vi "ZSLIM_OP100_LabelPrint.vi"(7 "Cluster":T1, 8 "errin":errorcluster) -> (0 "error out":errorcluster caption="errout")   [LabVIEW 2020]
uses:
  <vilib>/httpClient/POSTBuffer.vi
  <vilib>/httpClient/LabVIEWHTTPClient.lvlib
panel:
  out "body":string caption="corps"
  out "headers":string caption="en-têtes"
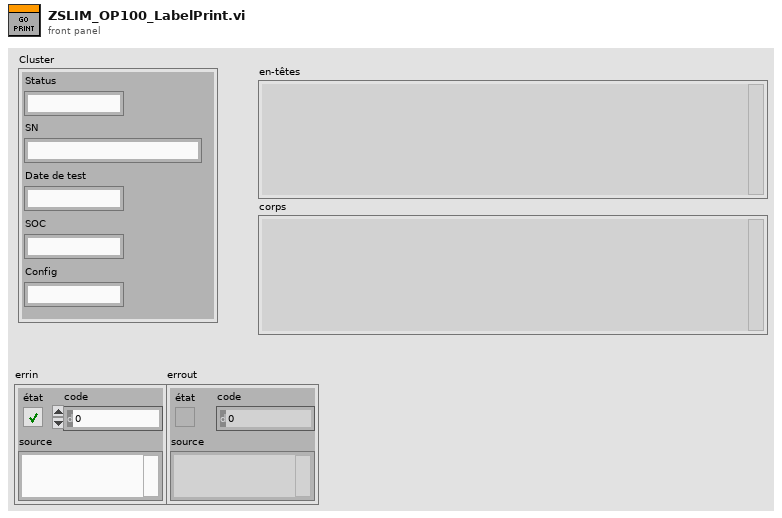
[diagram p1: front panel]
types:
  T1 = cluster{"Status":string, "SN":string, "Date de test":string, "SOC":string, "Config":string}
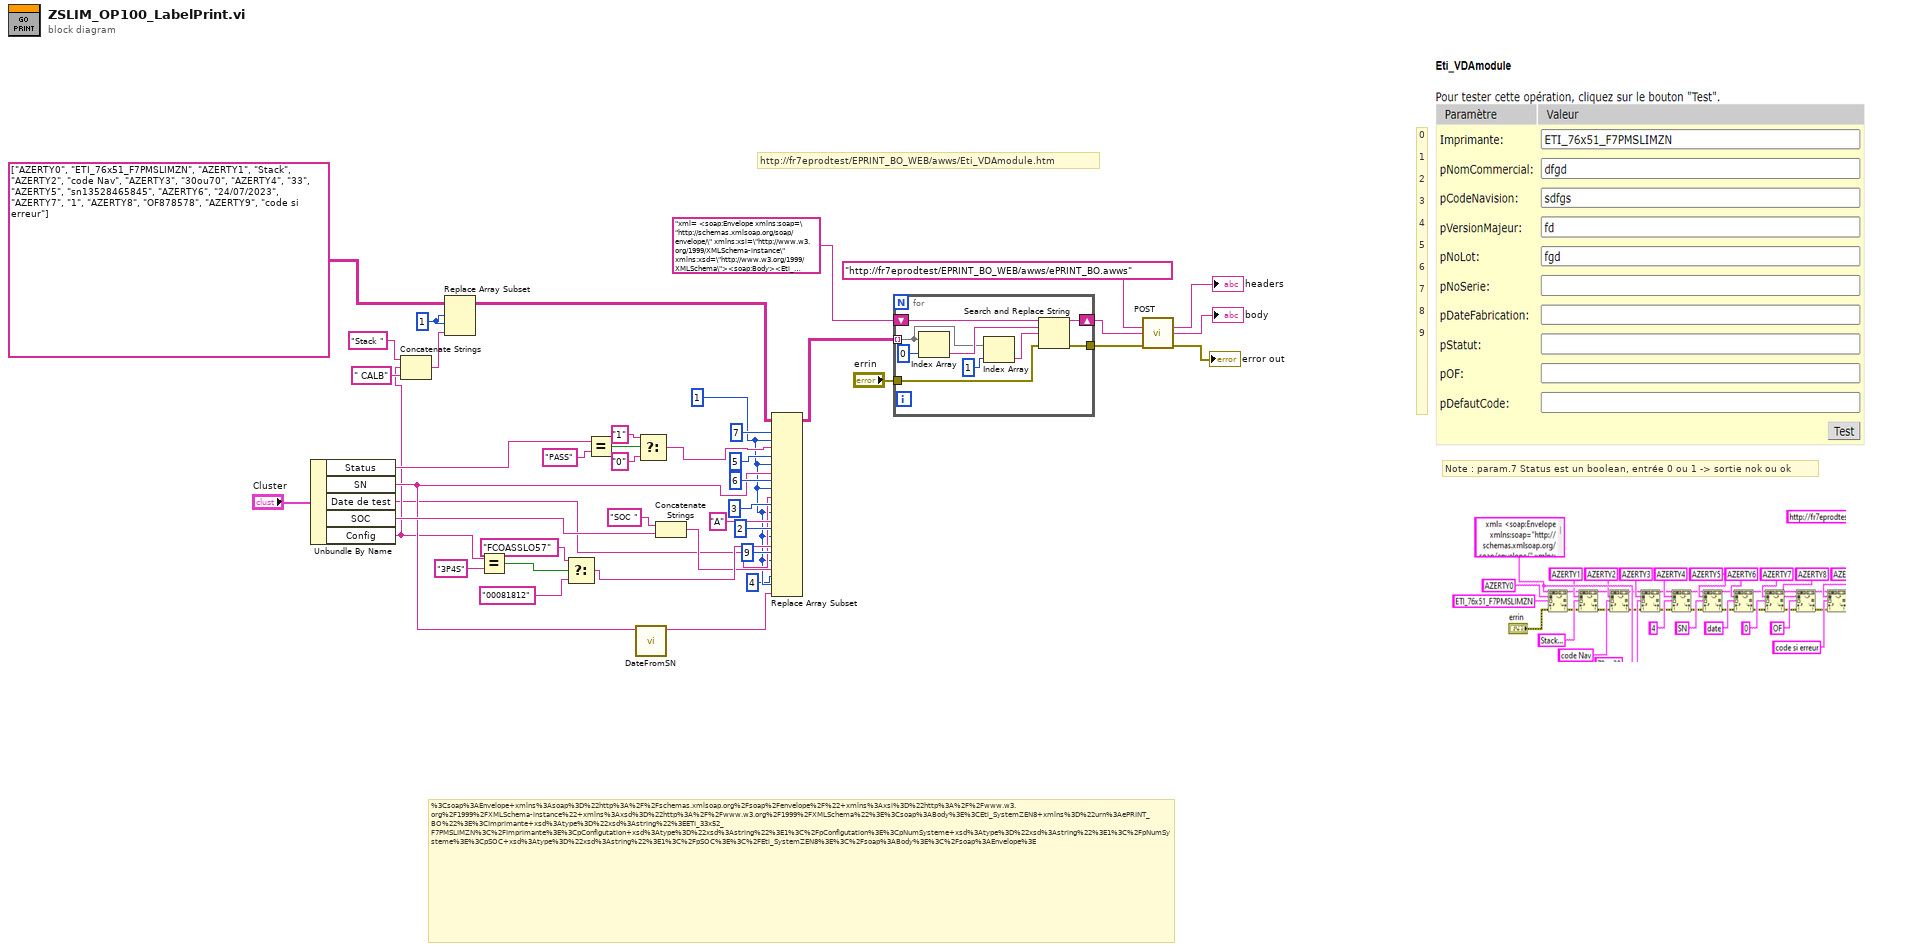
[diagram p0: block diagram]
diagram:
  w19 = 1 ("disabled index (col)")
  w2 = 1 ("disabled index (col)")
  # "http://fr7eprodtest/EPRINT_BO_WEB/awws/Eti_VDAmodule.htm"
  # "Note : param.7 Status est un boolean, entrée 0 ou 1 -> sortie nok ou ok"
  # "0\n\n1\n\n2\n\n3\n\n4\n\n5\n\n6\n\n7\n\n8\n\n9"
  # "%3Csoap%3AEnvelope+xmlns%3Asoap%3D%22http%3A%2F%2Fschemas.xmlsoap.org%2Fsoap%2Fenvelope%2F%22+xmlns%3Axsi%3D%22http%3A%2F%2Fwww.w3.org%2F1999%2FXMLSchema-instance%22+xmlns%3Axsd%3D%22http%3A%2F%2Fwww.w3.org%2F1999%2FXMLSchema%22%3E%3Csoap%3ABody%3E%3CEti_SystemZEN8+xmlns%3D%22urn%3AePRINT_BO%22%3E%3CImprimante+xsd%3Atype%3D%22xsd%3Astring%22%3EETI_33x52_F7PMSLIMZN%3C%2FImprimante%3E%3CpConfigutation+xsd%3Atype%3D%22xsd%3Astring%22%3E1%3C%2FpConfigutation%3E%3CpNumSysteme+xsd%3Atype%3D%22xsd%3Astring%22%3E1%3C%2FpNumSysteme%3E%3CpSOC+xsd%3Atype%3D%22xsd%3Astring%22%3E1%3C%2FpSOC%3E%3C%2FEti_SystemZEN8%3E%3C%2Fsoap%3ABody%3E%3C%2Fsoap%3AEnvelope%3E"
  n1 = Unbundle By Name("Cluster") -> ("Status"=w21:string, "SN"=w15:string, "Date de test"=w4:string, "SOC"=w20:string, "Config"=w13:string)
  n2 = Concatenate Strings("Stack " ("string"), w13, " CALB" ("string")) -> (w16:string)
  n3 = Replace Array Subset(array=string[][] [["AZERTY0", "ETI_76x51_F7PMSLIMZN"], ["AZERTY1", "Stack"], ["AZERTY2", "code Nav"], ["AZERTY3", "30ou70"], ["AZERTY4", "33"], ["AZERTY5", "sn13528465845"], ["AZERTY6", "24/07/2023"], ["AZERTY7", "1"], ["AZERTY8", "OF878578"], ["AZERTY9", "code si erreur"]], new element=w16, index (row)=w19, index (col)=w19) -> (w23:string[][])
  n4 = Equal?(x=w13, y="3P4S") -> (x = y?=w11:bool)
  n5 = Select(t="FCOASSLO57" ("y"), s=w11, f="00081812" ("y")) -> (s? t:f=w8:string)
  n6 = Equal?(x=w21, y="PASS") -> (x = y?=w34:bool)
  n7 = call "DateFromSN.vi"("SN"=w15) -> ("Date de fab"=w3:string)  [unwired: 10 in]
  n8 = Select(t="1" ("y"), s=w34, f="0") -> (s? t:f=w28:string)
  n9 = Concatenate Strings("SOC " ("string"), w20) -> (w5:string)
  n10 = Replace Array Subset(array=w23, new element #1=w28, index (row) #1=7 ("index (row)"), index (col) #1=w2, new element #2=w15, index (row) #2=5 ("disabled index (row)"), index (col) #2=w2, new element #3=w4, index (row) #3=6 ("disabled index (row)"), index (col) #3=w2, new element #4="A" ("new element/subarray"), index (row) #4=3 ("disabled index (row)"), index (col) #4=w2, new element #5=w8, index (row) #5=2 ("disabled index (row)"), index (col) #5=w2, new element #6=w5, index (row) #6=9 ("index (row)"), index (col) #6=w2, new element #7=w3, index (row) #7=4 ("disabled index (col)"), index (col) #7=w2) -> (w31:string[][])
  n11 = for {
    tunnel: w31 -> [w48] mode=indexing
    shift-right: [w51] -> w38
    shift-left: "xml= <soap:Envelope xmlns:soap=\"http://schemas.xmlsoap.org/soap/envelope/\" xmlns:xsi=\"http://www.w3.org/1999/XMLSchema-instance\" xmlns:xsd=\"http://www.w3.org/1999/XMLSchema\"><soap:Body><Eti_VDAmodule xmlns=\"urn:ePRINT_BO\"><Imprimante xsd:type=\"xsd:string\">AZERTY0</Imprimante><pNomCommercial xsd:type=\"xsd:string\">AZERTY1</pNomCommercial><pCodeNavision xsd:type=\"xsd:string\">AZERTY2</pCodeNavision><pVersionMajeur xsd:type=\"xsd:string\">AZERTY3</pVersionMajeur><pNoLot xsd:type=\"xsd:string\">AZERTY4</pNoLot><pNoSerie xsd:type=\"xsd:string\">AZERTY5</pNoSerie><pDateFabrication xsd:type=\"xsd:string\">AZERTY6</pDateFabrication><pStatut xsd:type=\"xsd:string\">AZERTY7</pStatut><pOF xsd:type=\"xsd:string\">AZERTY8</pOF><pDefautCode xsd:type=\"xsd:string\">AZERTY9</pDefautCode></Eti_VDAmodule></soap:Body></soap:Envelope>" ("buffer") -> [w52]
    tunnel: "errin" -> [w45]
    tunnel: [w44] -> w36
    n12 = Index Array(array=w48, index=0) -> (element=w50:string)
    n13 = Index Array(array=w48, index=1) -> (element=w46:string)
    n14 = Search and Replace String(input string=w52, search string=w50, replace string=w46, error in=w45) -> (result string=w51:string, error out=w44:errorcluster)  [unwired: 4 in, 2 out]
  }
  n15 = call-poly <vilib>:"POST.vi"("url"="http://fr7eprodtest/EPRINT_BO_WEB/awws/ePRINT_BO.awws", "buffer"=w38, "error in (no error)"=w36) -> ("headers"=→"headers":string, "body"=→"body":string, "error out"=→"error out":errorcluster)  [unwired: 9 in, 1 out]
